vi "Replace Spec Char string.vi"(8 "error in (no error)":errorcluster, 9 "SOH":i32, 10 "search string":string, 11 "String":string) -> (0 "error out":errorcluster, 3 "result string":string)   [LabVIEW 2016]
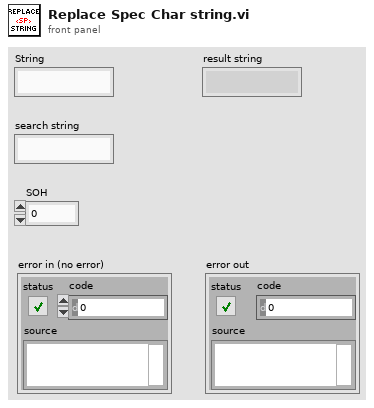
[diagram p1: front panel]
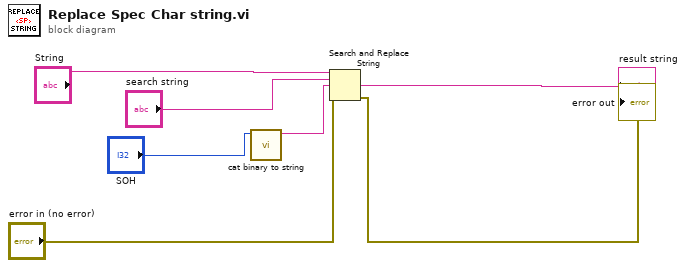
[diagram p0: block diagram]
diagram:
  n1 = call "cat binary to string.vi"("ETX"="SOH") -> ("String out"=w4:string)  [unwired: 10 in]
  n2 = Search and Replace String(input string="String", search string="search string", replace string=w4, error in="error in (no error)") -> (result string=→"result string":string, error out=→"error out":errorcluster)  [unwired: 4 in, 2 out]
